vi "get_temp_K.vi"(0 "VISA resource name":refnum<visa-resource-name>, 11 "error in (no error)":errorcluster) -> (4 "VISA resource name out":refnum<visa-resource-name>, 13 "Cold Head Temperature / K":dbl format="%.4f", 15 "error out":errorcluster)   [LabVIEW 2023]
uses:
  <instrlib>/Lake Shore 336/Lake Shore 336.lvlib
  <instrlib>/Lake Shore 336/Public/Data/Sensor Data (Single Reading).vi
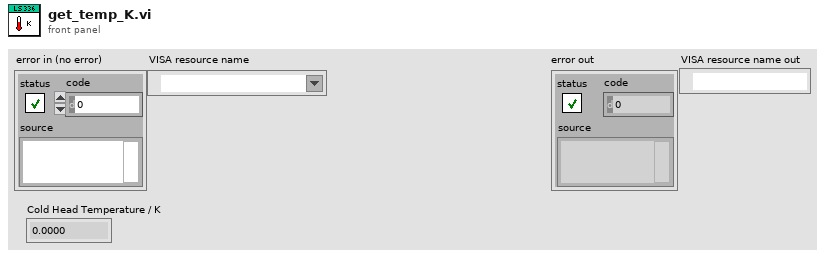
[diagram p1: front panel]
types:
  T1 = cluster{"Baud Rate":u32, "Parity":u16, "Data Bits":u16, "Stop Bits":u16, "Flow Control":u16}
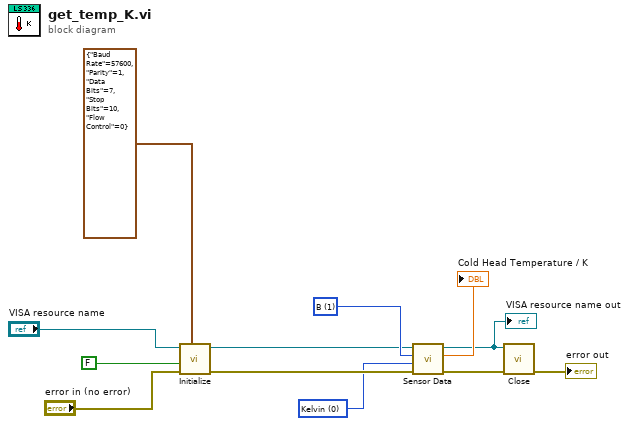
[diagram p0: block diagram]
diagram:
  w5 = u16 0 items=["Kelvin", "Celsius", "Sensor Units"] ("Data Source (0:Kelvin)")
  w10 = u16 1 items=["A", "B", "C", "D"] ("Input (0:A)")
  n1 = call <instrlib>:"Initialize.vi"("Serial Configuration"=T1 {"Baud Rate"=57600, "Parity"=1, "Data Bits"=7, "Stop Bits"=10, "Flow Control"=0}, "error in (no error)"="error in (no error)", "Reset (True)"=FALSE, "VISA resource name"="VISA resource name") -> ("error out"=w7:errorcluster, "VISA resource name out"=w8:refnum<visa-resource-name>)  [unwired: 6 in]
  n2 = call-poly <instrlib>:"Sensor Data.vi"("error in (no error)"=w7, "Data Source (0:Kelvin)"=w5, "Input (0:A)"=w10, "VISA resource name"=w8) -> ("error out"=w4:errorcluster, "Sensor Data"=→"Cold Head Temperature / K":dbl, "VISA resource name out"=w6:refnum<visa-resource-name>)  [unwired: 5 in]
  "VISA resource name out" <- w6
  n3 = call <instrlib>:"Close.vi"("error in (no error)"=w4, "VISA resource name"=w6) -> ("error out"=→"error out":errorcluster)  [unwired: 9 in]
